vi "Setup Statically-Linked subWorkers.vi"(8 "error in":errorcluster, 11 "subWorker Level 1 in":refnum<class "subWorker Level 1.lvclass">) -> (0 "error out":errorcluster, 3 "subWorker Level 1 out":refnum<class "subWorker Level 1.lvclass">)   [LabVIEW 2017, in "subWorker Level 1.lvclass"]
doc: "This VI performs a setup of all the statically-linked subWorkers that belong to the Worker that owns this VI. This VI must be called <b>before</b> any statically-linked subWorkers are called."
uses:
  subWorker Level 1.lvclass
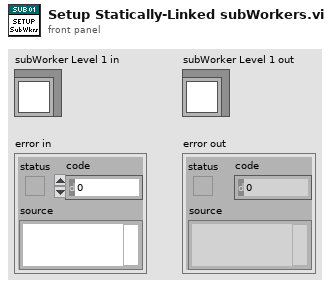
[diagram p1: front panel]
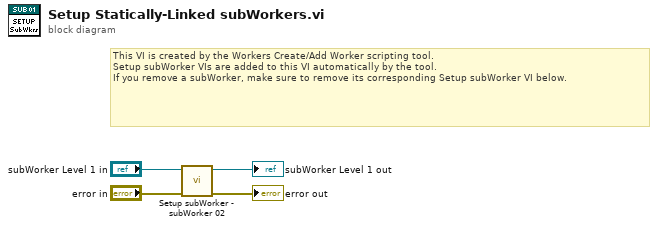
[diagram p0: block diagram]
diagram:
  # "This VI is created by the Workers Create/Add Worker scripting tool.\nSetup subWorker VIs are added to this VI automatically by the tool.\nIf you remove a subWorker, make sure to remove its corresponding Setup subWorker VI below."
  n1 = call "Setup subWorker - subWorker 02.vi"("error in"="error in", "subWorker Level 1 in"="subWorker Level 1 in") -> ("error out"=→"error out":errorcluster, "subWorker Level 1 out"=→"subWorker Level 1 out":refnum<class "subWorker Level 1.lvclass">)  [unwired: 8 in]
